vi "1-Convert Temperature.vi"() -> ()   [LabVIEW 2014]
panel:
  out "Temp (C)":i16
  in  "Temp (F)":i16
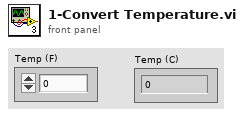
[diagram p1: front panel]
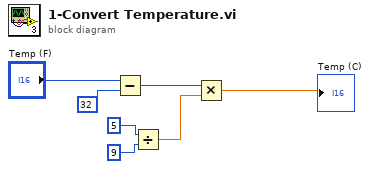
[diagram p0: block diagram]
diagram:
  n1 = Subtract(x="Temp (F)", y=32) -> (x-y=w2:i32)
  n2 = Divide(x=5, y=9) -> (x/y=w3:dbl)
  n3 = Multiply(x=w2, y=w3) -> (x*y=→"Temp (C)":dbl)
